vi "Write StartMarker.vi"(8 "error in (no error)":errorcluster, 10 "StartMarker":string="START", 11 "TCP_Server_Connection_Handler in":refnum<class "TCP_Server_Connection_Handler.lvclass">) -> (0 "error out":errorcluster, 3 "TCP_Server_Connection_Handler out":refnum<class "TCP_Server_Connection_Handler.lvclass">)   [LabVIEW 2023, in "TCP_Server_Connection_Handler.lvlib" / "TCP_Server_Connection_Handler.lvclass"]
uses:
  TCP_Server_Connection_Handler.lvclass
  TCP_Server_Connection_Handler.lvclass/TCP_Server_Connection_Handler.ctl
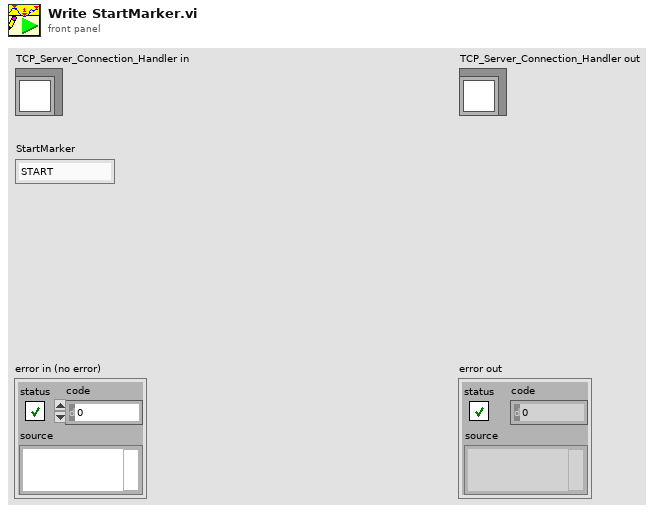
[diagram p1: front panel]
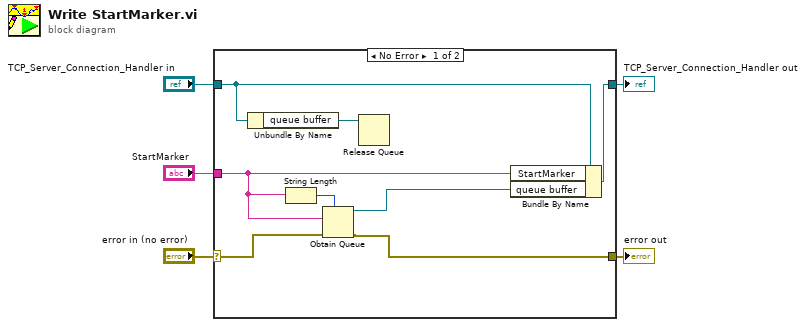
[diagram p0: block diagram]
diagram:
  n1 = case shown="No Error" "error in (no error)" {
    selector: "error in (no error)" -> [w8 w14]
    tunnel: [w7 w14] -> w4
    tunnel: [w13 w15] -> w2
    tunnel: "TCP_Server_Connection_Handler in" -> [w12 w15]
    tunnel: "StartMarker" -> [w9 _]
    frame No Error {
      n2 = Unbundle By Name(w12) -> ("queue buffer"=w11:refnum<queue>)
      n3 = String Length(string=w9) -> (length=w10:i32)
      n4 = Obtain Queue(max queue size (-1, unlimited)=w10, element data type=w9, error in (no error)=w8) -> (queue out=w6:refnum<queue>, error out=w7:errorcluster)  [unwired: 2 in, 1 out]
      n5 = Release Queue(queue=w11) -> ()  [unwired: 2 in, 3 out]
      n6 = Bundle By Name(cluster=w12, "StartMarker"=w9, "queue buffer"=w6) -> (w13:refnum<class "TCP_Server_Connection_Handler.lvclass">)
    }
    frame Error {
    }
  }
  "error out" <- w4
  "TCP_Server_Connection_Handler out" <- w2
